vi "DataLog Mirror Tag.vi"(0 "local db":string, 7 "tag":string, 11 "error in (no error)":errorcluster) -> (4 "mirrored values":dbl, 15 "error out":errorcluster)   [LabVIEW 2012]
doc: "Mirror the new data of a tag from a remote database to the mirrored local database."
uses:
  typedefs/t_DataLog Mirror State Methods.ctl
  typedefs/t_DataLog Mirror Served Methods.ctl
  typedefs/t_DataLog Databases Methods.ctl
  typedefs/t_DataLog Tag Info List Methods.ctl
  glb_DataLog MCVD.vi
panel:
  # "If you find that LabVIEW is stuck\nwhen calling this VI, you've likely\nmirrored a mirrored database such\nthat both are managed by the same\nserver runtime.\n\nOf course, that's useless, but maybe\nyou did it as a test. Anyways, it does\nnot work because LabVIEW will block\nbecause of a recursion deadlock on\nthis VI.\n\nMirroring a mirrored database\nbetween different server runtimes\nworks just fine."
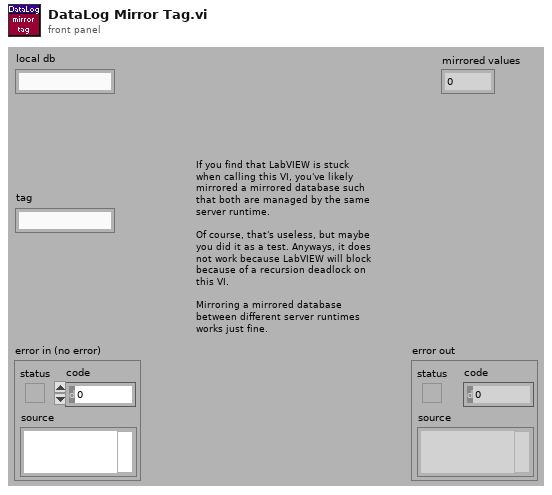
[diagram p1: front panel]
types:
  T1 = typedef "t_DataLog Tag Info List Methods.ctl" = enum16{"initialize", "create", "create empty", "rename", "delete", "test tag", "get", "get by name", "get default", "get list", "get path", "get subsets", "set subsets", "set config", "set capacity", "#tags", "go live", "set unlocked", "set mirrored"}
  T2 = typedef "t_DataLog Databases Methods.ctl" = enum16{"initialize", "get ref", "get names", "cleanup"}
  T3 = typedef "t_DataLog Mirror Served Methods.ctl" = enum16{"log info", "read range", "strsize", "read str"}
  T4 = typedef "t_DataLog Mirror State Methods.ctl" = enum16{"add db", "check db", "set", "get", "unset", "clear"}
  T5 = enum16{"deny read/write", "deny write-only", "deny none"}
  T6 = enum16{"read/write", "read-only", "write-only", "write-only (truncate)"}
  T7 = typedef "DataLog Mirror_srv.ctl" = refnum<vi>
  T8 = typedef "t_DataLog Database Info Pane.ctl" = refnum<vi>
  T9 = typedef "t_DataLog Tag Config.ctl" = cluster{"name":string, "unit":string, "temporal":T10, "value":T11, "index":i32, "capacity":i32, "is meta?":bool, "mincapacity":i32, "deadband":dbl, "limit delay":dbl, "format":T12, "precision":u8, "undefine":bool, "update":bool, "update period":u16, "expression":string, "description":string, "logging algorithm":T13, "logging parameters":dbl[]}
  T10 = typedef "t_DataLog Temporal Types.ctl" = enum16{"set&hold", "sample", "event"}
  T11 = typedef "t_DataLog Value Types.ctl" = enum16{"number", "string"}
  T12 = typedef "t_DataLog Numerical Format.ctl" = enum8{"fractional", "exponential", "engineering"}
  T13 = typedef "t_DataLog Logging Algorithms.ctl" = enum16{"nothing", "changes", "everything", "every Nth", "time threshold", "value threshold + prior", "t or v threshold", "t or v threshold + prior"}
  T14 = typedef "t_DataLog Point.ctl" = cluster{"time":dbl, "value":dbl}
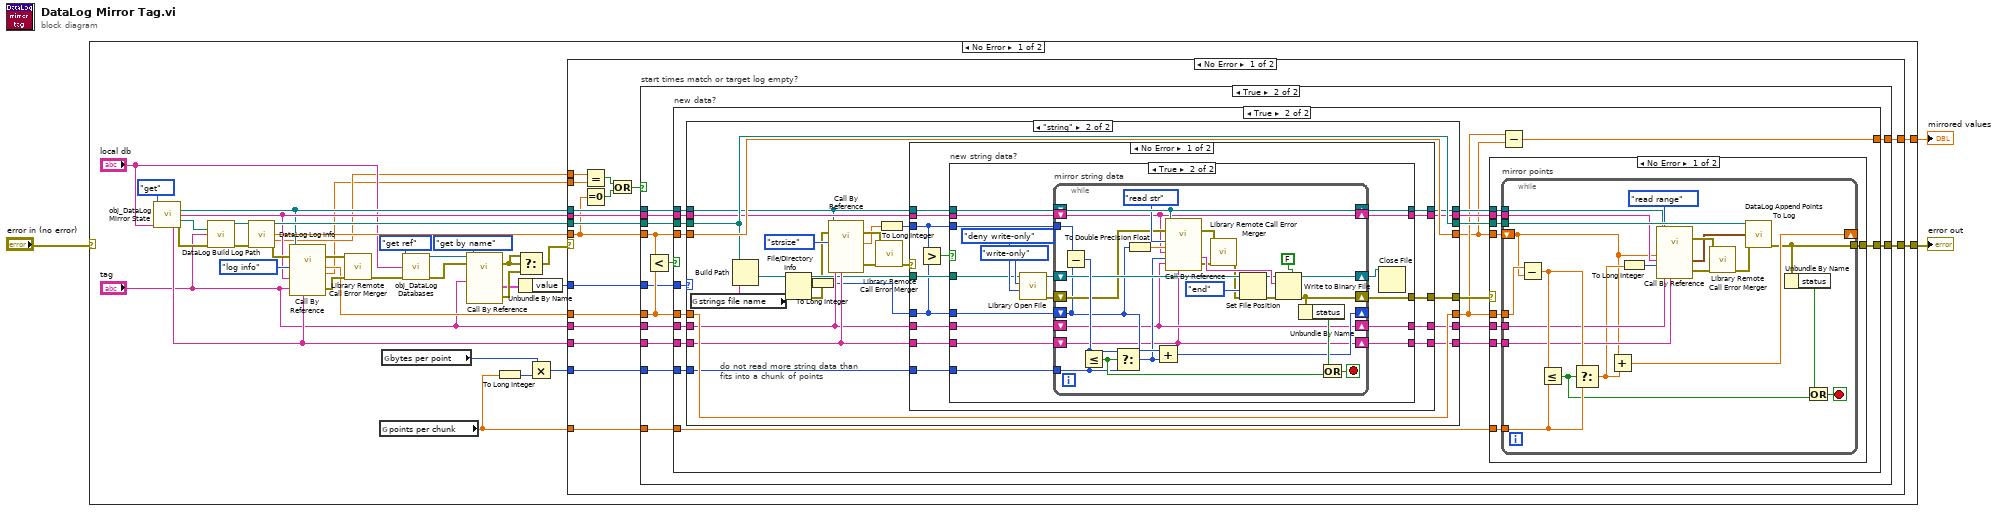
[diagram p0: block diagram]
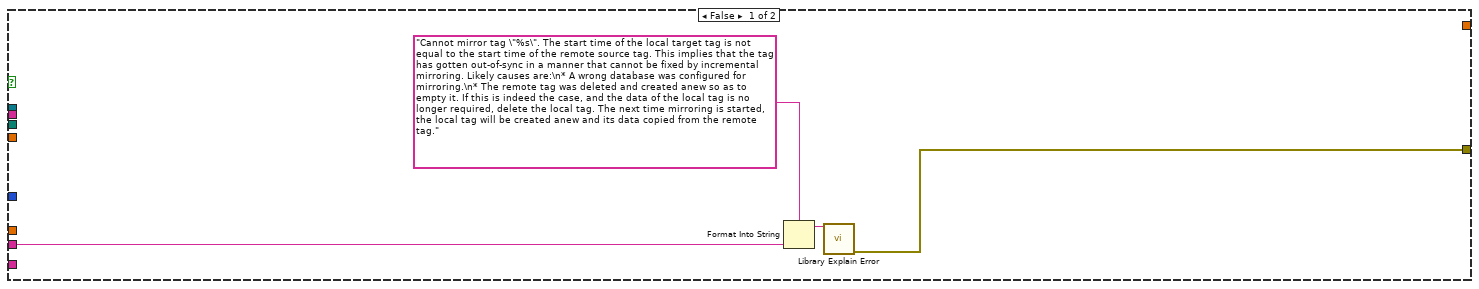
[diagram p2: hidden frame]
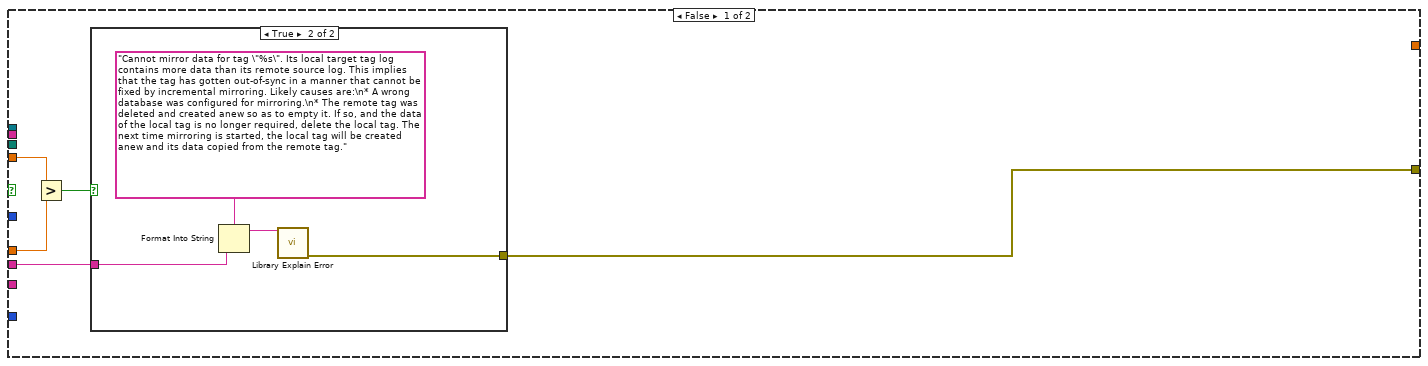
[diagram p3: hidden frame]
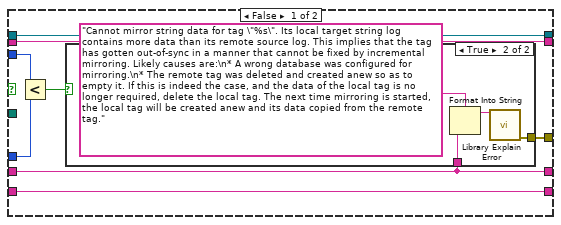
[diagram p6: hidden frame]
diagram:
  n1 = case shown="No Error" "error in (no error)" {
    selector: "error in (no error)" -> [_ w242]
    tunnel: [w30 w242] -> w2
    tunnel: [w4 _] -> w1
    frame No Error {
      n2 = call "obj_DataLog Mirror State.vi"("method"=t_DataLog_Mirror_State_Methods."get", "local db"="local db") -> ("mirror out"=w25:T7, "certificate out"=w26:string, "db path out"=w34:path, "remote db out"=w23:string, "get error"=w24:errorcluster)  [unwired: 8 in, 1 out]
      n3 = call "DataLog Build Log Path.vi"("database path"=w34, "tag"="tag", "error in (no error)"=w24) -> ("tag log directory"=w32:path, "error out"=w33:errorcluster)  [unwired: 11 in]
      n4 = call "DataLog Log Info.vi"("tag log directory"=w32, "error in (no error)"=w33) -> ("dup tag log directory"=w27:path, "size"=w29:dbl, "start time"=w6:dbl, "error out"=w31:errorcluster)  [unwired: 10 in]
      n5 = call-by-ref "?"(reference=w25, error in=w31, "method"=t_DataLog_Mirror_Served_Methods."log info", "certificate"=w26, "tag"="tag", "database"=w23) -> (error out=w37:errorcluster, "size"=w28:dbl, "start time"=w5:dbl, 15:"error out"=w36:errorcluster)  [unwired: 7 in, 3 out]
      n6 = call "Library Remote Call Error Merger.vi"("call by reference node error"=w37, "called VI error (no error)"=w36) -> ("error out"=w19:errorcluster)  [unwired: 13 in]
      n7 = global read "glb_DataLog MCVD.vi" "points per chunk"() -> (w21:dbl)
      n8 = global read "glb_DataLog MCVD.vi" "bytes per point"() -> (w22:i32)
      n9 = call "obj_DataLog Databases.vi"("method"=t_DataLog_Databases_Methods."get ref", "database (current)"="local db", "error in (no error)"=w19) -> ("database ref"=w16:T8, "error out"=w15:errorcluster)  [unwired: 10 in, 1 out]
      n10 = call-by-ref "?"(reference=w16, error in=w15, "method"=t_DataLog_Tag_Info_List_Methods."get by name", "tag or base tag"="tag") -> (error out=w14:errorcluster, "tag config out"=w10:T9, 15:"error out"=w13:errorcluster)  [unwired: 7 in, 6 out]
      n11 = To Long Integer(number=w21) -> (32bit integer=w20:i32)
      n12 = Select(t=w14, s=w14, f=w13) -> (s? t:f=w11:errorcluster)
      n13 = Unbundle By Name(w10) -> ("value"=w9:T11)
      n14 = Multiply(x=w22, y=w20) -> (x*y=w8:i32)
      n15 = case shown="No Error" w11 {
        selector: w11 -> [_ w241]
        tunnel: [w50 w241] -> w30
        tunnel: w29 -> [w45 _]
        tunnel: w28 -> [w53 _]
        tunnel: w27 -> [w55 _]
        tunnel: w26 -> [w49 _]
        tunnel: w23 -> [w48 _]
        tunnel: "tag" -> [w51 _]
        tunnel: w25 -> [w54 _]
        tunnel: w21 -> [w52 _]
        tunnel: w9 -> [w47 _]
        tunnel: w8 -> [w46 _]
        tunnel: w6 -> [w44 _]
        tunnel: w5 -> [w43 _]
        tunnel: [w39 _] -> w4
        frame No Error {
          n16 = Equal?(x=w44, y=w43) -> (x = y?=w41:bool)
          n17 = Equal To 0?(x=w45) -> (x = 0?=w42:bool)
          n18 = Or(x=w41, y=w42) -> (x .or. y?=w40:bool)
          n19 = case "start times match or target log empty?" shown="True" w40 {
            tunnel: w45 -> [_ w71]
            tunnel: w55 -> [_ w70]
            tunnel: w54 -> [_ w69]
            tunnel: w53 -> [_ w68]
            tunnel: w52 -> [_ w67]
            tunnel: w51 -> [w57 w66]
            tunnel: [w56 w65] -> w50
            tunnel: w49 -> [_ w64]
            tunnel: w48 -> [_ w63]
            tunnel: w47 -> [_ w62]
            tunnel: w46 -> [_ w61]
            tunnel: [_ w60] -> w39
            frame False {
              n20 = Format Into String(format string="Cannot mirror tag \"%s\". The start time of the local target tag is not equal to the start time of the remote source tag. This implies that the tag has gotten out-of-sync in a manner that cannot be fixed by incremental mirroring. Likely causes are:\n* A wrong database was configured for mirroring.\n* The remote tag was deleted and created anew so as to empty it. If this is indeed the case, and the data of the local tag is no longer required, delete the local tag. The next time mirroring is started, the local tag will be created anew and its data copied from the remote tag.", w57) -> (resulting string=w59:string)  [unwired: 2 in, 1 out]
              n21 = call "Library Explain Error.vi"("explanation prefix (none)"=w59) -> ("explained error"=w56:errorcluster)  [unwired: 14 in]
            }
            frame True {
              n22 = Less?(x=w71, y=w68) -> (x < y?=w72:bool)
              n23 = case "new data?" shown="True" w72 {
                tunnel: w71 -> [w77 w86]
                tunnel: w70 -> [_ w95]
                tunnel: w69 -> [_ w99]
                tunnel: w68 -> [w76 w93]
                tunnel: w67 -> [_ w88]
                tunnel: w66 -> [w74 w91]
                tunnel: [w73 w101] -> w65
                tunnel: w64 -> [_ w96]
                tunnel: w63 -> [_ w90]
                tunnel: w62 -> [_ w100]
                tunnel: w61 -> [_ w87]
                tunnel: [_ w82] -> w60
                frame False {
                  n24 = Greater?(x=w77, y=w76) -> (0:w75:bool)
                  n25 = case shown="True" w75 {
                    tunnel: w74 -> [_ w81]
                    tunnel: [_ w78] -> w73
                    frame False {
                    }
                    frame True {
                      n26 = Format Into String(format string="Cannot mirror data for tag \"%s\". Its local target tag log contains more data than its remote source log. This implies that the tag has gotten out-of-sync in a manner that cannot be fixed by incremental mirroring. Likely causes are:\n* A wrong database was configured for mirroring.\n* The remote tag was deleted and created anew so as to empty it. If so, and the data of the local tag is no longer required, delete the local tag. The next time mirroring is started, the local tag will be created anew and its data copied from the remote tag.", w81) -> (resulting string=w79:string)  [unwired: 2 in, 1 out]
                      n27 = call "Library Explain Error.vi"("explanation prefix (none)"=w79) -> ("explained error"=w78:errorcluster)  [unwired: 14 in]
                    }
                  }
                }
                frame True {
                  n28 = case shown="\"string\"" w100 {
                    tunnel: [w108 w130] -> w98
                    tunnel: w99 -> [w108 w122]
                    tunnel: w96 -> [w107 w129]
                    tunnel: [w107 w128] -> w97
                    tunnel: w95 -> [w106 w131]
                    tunnel: [w106 w131] -> w94
                    tunnel: w93 -> [w105 w127]
                    tunnel: [w105 w127] -> w84
                    tunnel: w91 -> [w104 w118]
                    tunnel: [w104 w125] -> w92
                    tunnel: w90 -> [w103 w119]
                    tunnel: [w103 w124] -> w89
                    tunnel: w87 -> [_ w115]
                    tunnel: w86 -> [w102 w132]
                    tunnel: [w102 w132] -> w83
                    tunnel: [_ w126] -> w85
                    frame "number" {
                    }
                    frame "string" {
                      # "do not read more string data than\nfits into a chunk of points"
                      n29 = global read "glb_DataLog MCVD.vi" "strings file name"() -> (w133:string)
                      n30 = Build Path(base path=w131, name or relative path=w133) -> (appended path=w113:path)
                      n31 = File/Directory Info(path=w113) -> (path out=w114:path, size=w109:i64, error out=w112:errorcluster)  [unwired: 1 in, 4 out]
                      n32 = To Long Integer(number=w109) -> (32bit integer=w111:i32)
                      n33 = call-by-ref "?"(reference=w122, error in=w112, "method"=t_DataLog_Mirror_Served_Methods."strsize", "tag"=w118, "database"=w119) -> (error out=w121:errorcluster, "size"=w117:dbl, 15:"error out"=w120:errorcluster)  [unwired: 8 in, 4 out]
                      n34 = call "Library Remote Call Error Merger.vi"("call by reference node error"=w121, "called VI error (no error)"=w120) -> ("error out"=w110:errorcluster)  [unwired: 13 in]
                      n35 = To Long Integer(number=w117) -> (32bit integer=w116:i32)
                      n36 = case shown="No Error" w110 {
                        selector: w110 -> [_ w205]
                        tunnel: [w147 w209] -> w130
                        tunnel: w129 -> [w146 w208]
                        tunnel: [w145 w208] -> w128
                        tunnel: [w144 w205] -> w126
                        tunnel: [w143 w207] -> w125
                        tunnel: [w142 w206] -> w124
                        tunnel: w122 -> [w141 w209]
                        tunnel: w119 -> [w140 w206]
                        tunnel: w118 -> [w139 w207]
                        tunnel: w116 -> [w136 _]
                        tunnel: w115 -> [w138 _]
                        tunnel: w114 -> [w137 _]
                        tunnel: w111 -> [w135 _]
                        frame No Error {
                          n37 = Greater?(x=w136, y=w135) -> (0:w134:bool)
                          n38 = case "new string data?" shown="True" w134 {
                            tunnel: [w155 w175] -> w147
                            tunnel: w146 -> [w154 w174]
                            tunnel: [w154 w173] -> w145
                            tunnel: [w152 w171] -> w144
                            tunnel: [w151 w170] -> w143
                            tunnel: [w153 w169] -> w142
                            tunnel: w141 -> [w155 w168]
                            tunnel: w140 -> [w153 w167]
                            tunnel: w139 -> [w151 w166]
                            tunnel: w136 -> [w150 w161]
                            tunnel: w138 -> [_ w165]
                            tunnel: w137 -> [_ w162]
                            tunnel: w135 -> [w149 w160]
                            frame False {
                              n39 = Less?(x=w150, y=w149) -> (x < y?=w148:bool)
                              n40 = case shown="True" w148 {
                                tunnel: [_ w157] -> w152
                                tunnel: w151 -> [_ w156]
                                frame False {
                                }
                                frame True {
                                n41 = Format Into String(format string="Cannot mirror string data for tag \"%s\". Its local target string log contains more data than its remote source log. This implies that the tag has gotten out-of-sync in a manner that cannot be fixed by incremental mirroring. Likely causes are:\n* A wrong database was configured for mirroring.\n* The remote tag was deleted and created anew so as to empty it. If this is indeed the case, and the data of the local tag is no longer required, delete the local tag. The next time mirroring is started, the local tag will be created anew and its data copied from the remote tag.", w156) -> (resulting string=w158:string)  [unwired: 2 in, 1 out]
                                n42 = call "Library Explain Error.vi"("explanation prefix (none)"=w158) -> ("explained error"=w157:errorcluster)  [unwired: 14 in]
                                }
                              }
                            }
                            frame True {
                              n43 = call "Library Open File.vi"("deny mode (deny none)"=T5."deny write-only" ("deny mode (2)"), "open mode (read/write)"=T6."write-only" ("open mode (0)"), "file path"=w162) -> ("error out"=w163:errorcluster, "refnum"=w164:refnum<file>)  [unwired: 3 in]
                              n44 = while "mirror string data" {
                                shift-right: [w194] -> w175
                                shift-left: w168 -> [w194]
                                shift-right: [w180] -> w173
                                shift-left: w174 -> [w180]
                                shift-right: [w202] -> w171
                                shift-left: w163 -> [w192]
                                shift-right: [w179] -> w170
                                shift-left: w166 -> [w179]
                                shift-right: [w178] -> w169
                                shift-left: w167 -> [w178]
                                shift-right: [w195] -> w172
                                shift-left: w164 -> [w197]
                                shift-right: [w196] -> _
                                shift-left: w160 -> [w190]
                                tunnel: w161 -> [w203]
                                tunnel: w165 -> [w184]
                                stop <- w201 stop-if-true
                                n45 = Subtract(x=w203, y=w190) -> (x-y=w198:i32)
                                n46 = Less Or Equal?(x=w198, y=w184) -> (x <= y?=w199:bool)
                                n47 = Select(t=w198, s=w199, f=w184) -> (s? t:f=w189:i32)
                                n48 = To Double Precision Float(number=w190) -> (double precision float=w191:dbl)
                                n49 = Add(x=w190, y=w189) -> (x+y=w196:i32)
                                n50 = call-by-ref "?"(reference=w194, error in=w192, "method"=t_DataLog_Mirror_Served_Methods."read str", "log index"=w191, "certificate"=w180, "amount"=w189, "tag"=w179, "database"=w178) -> (error out=w188:errorcluster, "string data"=w187:string, 15:"error out"=w186:errorcluster)  [unwired: 5 in, 4 out]
                                n51 = call "Library Remote Call Error Merger.vi"("call by reference node error"=w188, "called VI error (no error)"=w186) -> ("error out"=w185:errorcluster)  [unwired: 13 in]
                                n52 = Set File Position(refnum=w197, from (0:start)=enum16{"start", "end", "current"}."end" ("pos mode (0:2)"), error in=w185) -> (refnum out=w183:refnum<file>, error out=w182:errorcluster)  [unwired: 1 in]
                                n53 = Write to Binary File(file (use dialog)=w183, data=w187, error in=w182, 5:FALSE ("prepend array or string size? (T)")) -> (refnum out=w195:refnum<file>, error out=w202:errorcluster)  [unwired: 2 in, 1 out]
                                n54 = Unbundle By Name(w202) -> ("status"=w200:bool)
                                n55 = Or(x=w200, y=w199) -> (x .or. y?=w201:bool)
                              }
                              n56 = Close File(refnum=w172) -> ()  [unwired: 1 in, 2 out]
                            }
                          }
                        }
                        frame Error {
                        }
                      }
                    }
                  }
                  n57 = case shown="No Error" w85 {
                    selector: w85 -> [_ w240]
                    tunnel: w94 -> [w218 _]
                    tunnel: w98 -> [w217 _]
                    tunnel: w83 -> [w216 _]
                    tunnel: w84 -> [w215 _]
                    tunnel: w88 -> [w214 _]
                    tunnel: w92 -> [w210 _]
                    tunnel: [w213 w240] -> w101
                    tunnel: w97 -> [w212 _]
                    tunnel: w89 -> [w211 _]
                    frame No Error {
                      n58 = while "mirror points" {
                        tunnel: w218 -> [w239]
                        tunnel: w217 -> [w238]
                        shift-right: [w230] -> _
                        shift-left: w216 -> [w219]
                        tunnel: w215 -> [w236]
                        tunnel: w214 -> [w235]
                        tunnel: w211 -> [w229]
                        tunnel: w210 -> [w228]
                        tunnel: [w222] -> w213
                        tunnel: w212 -> [w220]
                        stop <- w232 stop-if-true
                        n59 = Subtract(x=w236, y=w219) -> (x-y=w234:dbl)
                        n60 = Less Or Equal?(x=w234, y=w235) -> (x <= y?=w233:bool)
                        n61 = Select(t=w234, s=w233, f=w235) -> (s? t:f=w227:dbl)
                        n62 = Add(x=w219, y=w227) -> (x+y=w230:dbl)
                        n63 = To Long Integer(number=w227) -> (32bit integer=w231:i32)
                        n64 = call-by-ref "?"(reference=w238, "method"=t_DataLog_Mirror_Served_Methods."read range", "log index"=w219, "certificate"=w220, "amount"=w231, "tag"=w228, "database"=w229) -> (error out=w226:errorcluster, "points"=w223:T14[], 15:"error out"=w225:errorcluster)  [unwired: 6 in, 4 out]
                        n65 = call "Library Remote Call Error Merger.vi"("call by reference node error"=w226, "called VI error (no error)"=w225) -> ("error out"=w224:errorcluster)  [unwired: 13 in]
                        n66 = call "DataLog Append Points To Log.vi"("tag log directory"=w239, "points"=w223, "error in (no error)"=w224) -> ("error out"=w222:errorcluster)  [unwired: 11 in, 1 out]
                        n67 = Unbundle By Name(w222) -> ("status"=w221:bool)
                        n68 = Or(x=w221, y=w233) -> (x .or. y?=w232:bool)
                      }
                    }
                    frame Error {
                    }
                  }
                  n69 = Subtract(x=w84, y=w83) -> (x-y=w82:dbl)
                }
              }
            }
          }
        }
        frame Error {
        }
      }
    }
    frame Error {
    }
  }
  "error out" <- w2
  "mirrored values" <- w1
